vi "setDilutionControls.vi"() -> ()   [LabVIEW 2011]
uses:
  bubblerDilution.ctl
panel:
  out "output cluster":T1
  in  "Ga bubbler In":T2={"Active"=FALSE, "main"={"Flow"=0.0, "Run"=FALSE, "Prep Ga"=FALSE, "Dilution"=FALSE, "Calculated"=0, "MFC2 flow"=10.0, "MFC3 flow"=100.0, "MFC1 flow"=0.0}} {"main"."MFC1 flow" format="%.4f"; "main"."MFC3 flow" format="%.1f"; "main"."MFC2 flow" format="%.2f"; "main"."Calculated" items=["Flow", "MFC1", "MFC2", "MFC3"]; "main"."Flow" format="%.2f"}
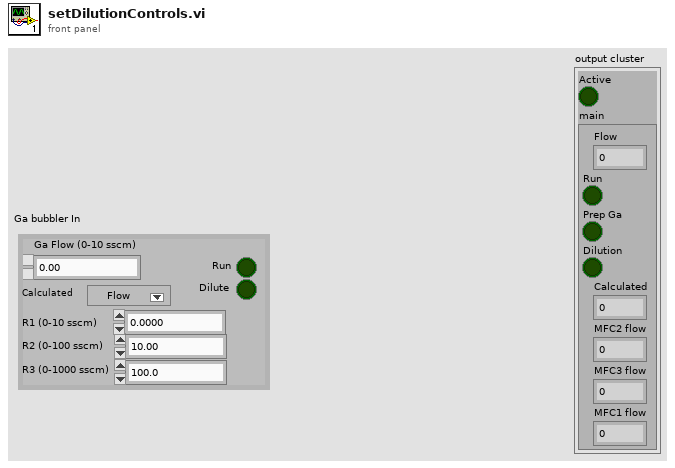
[diagram p1: front panel]
types:
  T1 = cluster{"Active":bool, "main":cluster{"Flow":dbl, "Run":bool, "Prep Ga":bool, "Dilution":bool, "Calculated":u16, "MFC2 flow":dbl, "MFC3 flow":dbl, "MFC1 flow":dbl}}
  T2 = typedef "bubblerDilution.ctl" = cluster{"Active":bool, "main":cluster{"Flow":dbl, "Run":bool, "Prep Ga":bool, "Dilution":bool, "Calculated":u16, "MFC2 flow":dbl, "MFC3 flow":dbl, "MFC1 flow":dbl}}
  T3 = enum8{"Enabled", "Disabled", "Disabled and Grayed Out"}
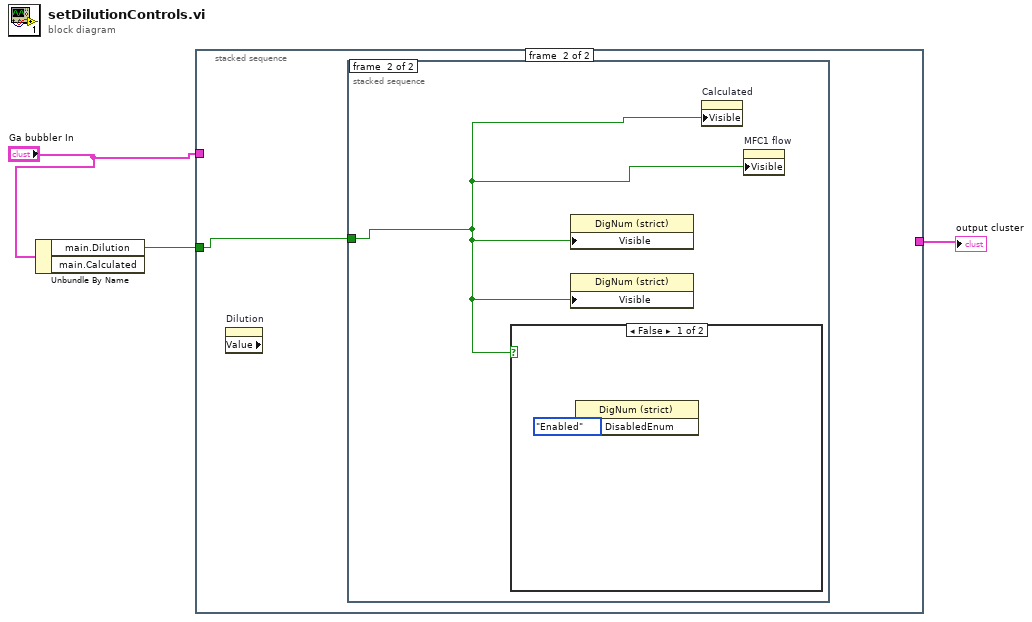
[diagram p0: block diagram]
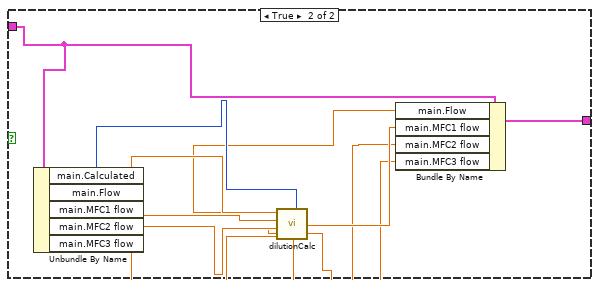
[diagram p3: hidden frame]
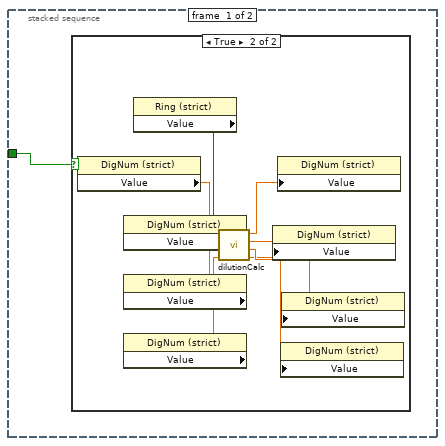
[diagram p4: hidden frame]
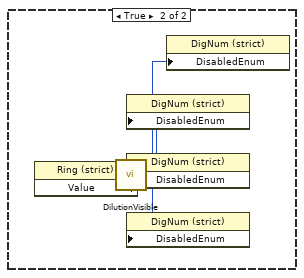
[diagram p6: hidden frame]
diagram:
  n1 = Unbundle By Name("Ga bubbler In") -> ("main.Dilution"=w2:bool)  [unwired: 1 out]
  n2 = stacked-sequence {
    tunnel: [w5 _] -> w3
    tunnel: w2 -> [w6 w18]
    tunnel: "Ga bubbler In" -> [w4 _]
    frame #0 {
      n3 = case shown="False" w6 {
        tunnel: [_ w17] -> w5
        tunnel: w4 -> [_ w7]
        frame False {
        }
        frame True {
          n4 = Unbundle By Name(w7) -> ("main.Calculated"=w16:u16, "main.Flow"=w15:dbl, "main.MFC1 flow"=w14:dbl, "main.MFC2 flow"=w13:dbl, "main.MFC3 flow"=w12:dbl)
          n5 = call "dilutionCalc.vi"("Calculated"=w16, "MFC3"=w12, "MFC2"=w13, "MFC1"=w14, "flow"=w15) -> ("MFC3 out"=w8:dbl, "MFC2 out"=w9:dbl, "MFC1 out"=w10:dbl, "flow out"=w11:dbl)  [unwired: 1 in]
          n6 = Bundle By Name(cluster=w7, "main.Flow"=w11, "main.MFC1 flow"=w10, "main.MFC2 flow"=w9, "main.MFC3 flow"=w8) -> (w17:T2)
        }
      }
    }
    frame #1 {
      n7 = property on="Dilution" class="Bool (strict)" props=["Value"]() -> ()  [unwired: 2 in, 3 out]
      n8 = stacked-sequence {
        tunnel: w18 -> [w19 w29]
        frame #0 {
          n9 = case shown="True" w19 {
            frame False {
            }
            frame True {
              n10 = property on="Property Node" class="DigNum (strict)"() -> ("Value"=w27:dbl)  [unwired: 2 in, 2 out]
              n11 = property on="Property Node" class="DigNum (strict)"() -> ("Value"=w26:dbl)  [unwired: 2 in, 2 out]
              n12 = property on="Property Node" class="DigNum (strict)"() -> ("Value"=w25:dbl)  [unwired: 2 in, 2 out]
              n13 = property on="Property Node" class="DigNum (strict)"() -> ("Value"=w24:dbl)  [unwired: 2 in, 2 out]
              n14 = property on="Property Node" class="Ring (strict)"() -> ("Value"=w28:u16)  [unwired: 2 in, 2 out]
              n15 = call "dilutionCalc.vi"("Calculated"=w28, "MFC3"=w24, "MFC2"=w25, "MFC1"=w26, "flow"=w27) -> ("MFC3 out"=w20:dbl, "MFC2 out"=w21:dbl, "MFC1 out"=w22:dbl, "flow out"=w23:dbl)  [unwired: 1 in]
              n16 = property on="Property Node" class="DigNum (strict)"("Value"=w22) -> ()  [unwired: 2 in, 2 out]
              n17 = property on="Property Node" class="DigNum (strict)"("Value"=w23) -> ()  [unwired: 2 in, 2 out]
              n18 = property on="Property Node" class="DigNum (strict)"("Value"=w20) -> ()  [unwired: 2 in, 2 out]
              n19 = property on="Property Node" class="DigNum (strict)"("Value"=w21) -> ()  [unwired: 2 in, 2 out]
            }
          }
        }
        frame #1 {
          n20 = case shown="False" w29 {
            frame False {
              n21 = property on="Property Node" class="DigNum (strict)"("DisabledEnum"=T3."Enabled" ("Disabled")) -> ()  [unwired: 2 in, 2 out]
            }
            frame True {
              n22 = property on="Property Node" class="Ring (strict)"() -> ("Value"=w31:u16)  [unwired: 2 in, 2 out]
              n23 = call "DilutionVisible.vi"("calculated"=w31) -> ("MFC3"=w35:u16, "MFC2"=w34:u16, "MFC1"=w33:u16, "flow"=w32:u16)  [unwired: 3 in]
              n24 = property on="Property Node" class="DigNum (strict)"("DisabledEnum"=w33) -> ()  [unwired: 2 in, 2 out]
              n25 = property on="Property Node" class="DigNum (strict)"("DisabledEnum"=w34) -> ()  [unwired: 2 in, 2 out]
              n26 = property on="Property Node" class="DigNum (strict)"("DisabledEnum"=w35) -> ()  [unwired: 2 in, 2 out]
              n27 = property on="Property Node" class="DigNum (strict)"("DisabledEnum"=w32) -> ()  [unwired: 2 in, 2 out]
            }
          }
          n28 = property on="Property Node" class="DigNum (strict)"("Visible"=w29) -> ()  [unwired: 2 in, 2 out]
          n29 = property on="Property Node" class="DigNum (strict)"("Visible"=w29) -> ()  [unwired: 2 in, 2 out]
          n30 = property on="Calculated" class="Ring (strict)"("Visible"=w29) -> ()  [unwired: 2 in, 2 out]
          n31 = property on="MFC1 flow" class="DigNum (strict)"("Visible"=w29) -> ()  [unwired: 2 in, 2 out]
        }
      }
    }
  }
  "output cluster" <- w3
